vi "Traps-10-06-2017.vi"(0 "d0Trap1":fxp<+/-,18,18> format="%.16g", 1 "heizenTrap1":bool, 2 "U_SPTrap1":fxp<+/-,26,5> format="%.23g", 3 "->Register":u32, 5 "d1Trap1":fxp<+/-,21,21> format="%.16g", 7 "Warten(uSec)":u16=5000, 9 "d0Trap2":fxp<+/-,18,18> format="%.16g", 11 "d1Trap2":fxp<+/-,21,21> format="%.16g", 12 "heizenTrap2":bool, 13 "U_SPTrap2":fxp<+/-,26,5> format="%.23g") -> (4 "U_MWTrap1":fxp<+/-,26,5> format="%.23g", 14 "Register->":u32, 15 "U_MWTrap2":fxp<+/-,26,5> format="%.23g")   [LabVIEW 2010]
uses:
  <vilib>/eio/EIONode/EIONode.xnode
  <vilib>/rvi/eio/nirviEIOImplementation/nirviEIOImplementation.xnode
  <vilib>/rvi/eio/common/nirviEmuClasses.ctl
  <vilib>/rvi/FXPMathLib/FxpAdd/XNode/nifxpmath_Add.xnode
  <vilib>/rvi/FXPMathLib/FxpAdd/subVIs/nifxpmath_Add_SimConfig.ctl
  <vilib>/fxp/LVFixedPointQuantizationPolicyTypeDef.ctl
  <vilib>/fxp/LVFixedPointOverflowPolicyTypeDef.ctl
  <vilib>/rvi/FXPMathLib/FxpDiv/XNode/nifxpmath_Div.xnode
  <vilib>/rvi/FXPMathLib/FxpDiv/subVIs/nifxpmath_Div_SimConfig.ctl
  <vilib>/rvi/FXPMathLib/FxpSub/XNode/nifxpmath_Sub.xnode
  <vilib>/rvi/FXPMathLib/FxpSub/subVIs/nifxpmath_Sub_SimConfig.ctl
  <vilib>/rvi/FXPMathLib/FxpMul/XNode/nifxpmath_Multiplier.xnode
  <vilib>/rvi/FXPMathLib/FxpMul/subVIs/nifxpmath_Mul_SimConfig.ctl
  <vilib>/rvi/eio/common/nirviEmuTemplateMethod_noerrors.vi
  <vilib>/rvi/FXPMathLib/FxpAdd/simVIs/DllFxpAddTemp_sub.vi
  <vilib>/rvi/FXPMathLib/FxpDiv/simVIs/DllFxpDivTemp_sub.vi
  <vilib>/rvi/FXPMathLib/FxpSub/simVIs/DllFxpSubTemp_sub.vi
  <vilib>/rvi/FXPMathLib/FxpMul/simVIs/DllFxpMulTemp_sub.vi
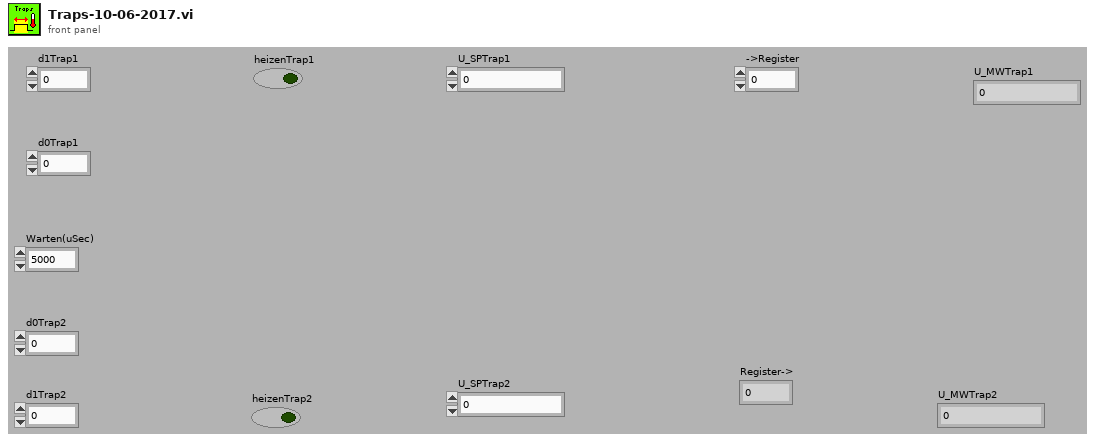
[diagram p1: front panel]
types:
  T1 = typedef "nirviEmuClasses.ctl" = enum16{"IO Read", "IO Write", "Method", "Property Read", "Property Write"}
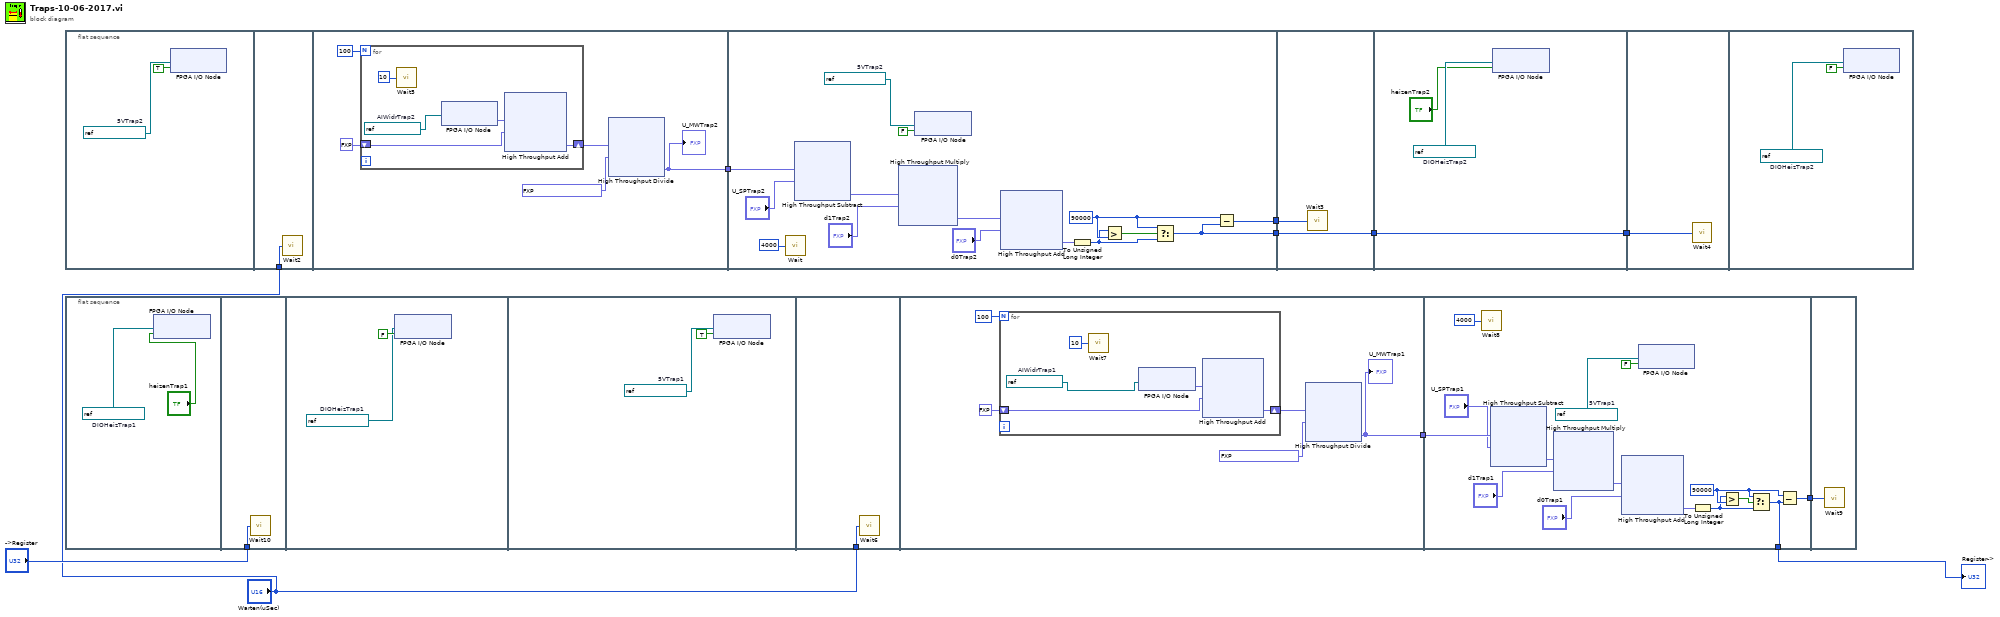
[diagram p0: block diagram]
diagram:
  n1 = flat-sequence {
    tunnel: "Warten(uSec)" -> [w24]
    tunnel: [w25] -> w9
    tunnel: w9 -> [w123]
    tunnel: [w115] -> w8
    tunnel: [w119] -> w7
    tunnel: [w225] -> w6
    tunnel: w8 -> [w225]
    tunnel: w7 -> [w224]
    tunnel: [w228] -> w5
    tunnel: w6 -> [w228]
    tunnel: w5 -> [w240]
    frame #0 {
      w11 = refnum<k21> "Mod6/DIO20"  # 5VTrap2
      n2 = xnode "FPGA I/O Node"("I/O Item"=TRUE, "FPGA I/O In"=w11) -> ()  [unwired: 1 out]
    }
    frame #1 {
      n3 = call "Wait2"("Count(uSec)"=w24) -> ()  [unwired: 1 out]
    }
    frame #2 {
      n4 = for {
        N: 100 -> [_]
        shift-right: [w58] -> w29
        shift-left: fxp<+/-,33,12> 0.0 ("x+y") -> [w59]
        w57 = refnum<k21> "Mod1/AI31"  # AIWidrTrap2
        n5 = call "Wait5"("Count(uSec)"=u8 10) -> ()  [unwired: 1 out]
        n6 = xnode "FPGA I/O Node"("FPGA I/O In"=w57) -> ("I/O Item"=w60:fxp<+/-,26,5>)  [unwired: 1 out]
        n7 = xnode "High Throughput Add"("x"=w60, "y"=w59) -> ("x+y"=w58:fxp<+/-,33,12>)
      }
      n8 = xnode "High Throughput Divide"("x"=w29, "y"=fxp<+/-,8,8> 100.0) -> ("x/y"=w25:fxp<+/-,26,5>)
      "U_MWTrap2" <- w25
    }
    frame #3 {
      w114 = refnum<k21> "Mod6/DIO20"  # 5VTrap2
      w117 = u32 90000 ("x")
      n9 = call "Wait"("Count(uSec)"=u16 4000) -> ()  [unwired: 1 out]
      n10 = xnode "High Throughput Subtract"("x"=w123, "y"="U_SPTrap2") -> ("x-y"=w122:fxp<+/-,26,5>)
      n11 = xnode "High Throughput Multiply"("x"=w122, "y"="d1Trap2") -> ("x*y"=w121:fxp<+/-,18,18>)
      n12 = xnode "FPGA I/O Node"("I/O Item"=FALSE, "FPGA I/O In"=w114) -> ()  [unwired: 1 out]
      n13 = xnode "High Throughput Add"("x"=w121, "y"="d0Trap2") -> ("x+y"=w120:fxp<+/-,18,18>)
      n14 = To Unsigned Long Integer(number=w120) -> (unsigned 32bit integer=w116:u32)
      n15 = Greater?(x=w116, y=w117) -> (0:w118:bool)
      n16 = Select(t=w117, s=w118, f=w116) -> (s? t:f=w115:u32)
      n17 = Subtract(x=w117, y=w115) -> (x-y=w119:u32)
    }
    frame #4 {
      n18 = call "Wait3"("Count(uSec)"=w224) -> ()  [unwired: 1 out]
    }
    frame #5 {
      w227 = refnum<k21> "Mod6/DIO18"  # DIOHeizTrap2
      n19 = xnode "FPGA I/O Node"("I/O Item"="heizenTrap2", "FPGA I/O In"=w227) -> ()  [unwired: 1 out]
    }
    frame #6 {
      n20 = call "Wait4"("Count(uSec)"=w240) -> ()  [unwired: 1 out]
    }
    frame #7 {
      w241 = refnum<k21> "Mod6/DIO18"  # DIOHeizTrap2
      n21 = xnode "FPGA I/O Node"("I/O Item"=FALSE, "FPGA I/O In"=w241) -> ()  [unwired: 1 out]
    }
  }
  n22 = flat-sequence {
    tunnel: "->Register" -> [w267]
    tunnel: "Warten(uSec)" -> [w294]
    tunnel: [w295] -> w4
    tunnel: w4 -> [w393]
    tunnel: [w389] -> w3
    tunnel: [w385] -> w2
    tunnel: w3 -> [w494]
    frame #0 {
      w255 = refnum<k21> "Mod6/DIO19"  # DIOHeizTrap1
      n23 = xnode "FPGA I/O Node"("I/O Item"="heizenTrap1", "FPGA I/O In"=w255) -> ()  [unwired: 1 out]
    }
    frame #1 {
      n24 = call "Wait10"("Count(uSec)"=w267) -> ()  [unwired: 1 out]
    }
    frame #2 {
      w268 = refnum<k21> "Mod6/DIO19"  # DIOHeizTrap1
      n25 = xnode "FPGA I/O Node"("I/O Item"=FALSE, "FPGA I/O In"=w268) -> ()  [unwired: 1 out]
    }
    frame #3 {
      w281 = refnum<k21> "Mod6/DIO21"  # 5VTrap1
      n26 = xnode "FPGA I/O Node"("I/O Item"=TRUE, "FPGA I/O In"=w281) -> ()  [unwired: 1 out]
    }
    frame #4 {
      n27 = call "Wait6"("Count(uSec)"=w294) -> ()  [unwired: 1 out]
    }
    frame #5 {
      n28 = for {
        N: 100 -> [_]
        shift-right: [w328] -> w299
        shift-left: fxp<+/-,33,12> 0.0 ("x+y") -> [w329]
        w327 = refnum<k21> "Mod1/AI30"  # AIWidrTrap1
        n29 = call "Wait7"("Count(uSec)"=u8 10) -> ()  [unwired: 1 out]
        n30 = xnode "FPGA I/O Node"("FPGA I/O In"=w327) -> ("I/O Item"=w330:fxp<+/-,26,5>)  [unwired: 1 out]
        n31 = xnode "High Throughput Add"("x"=w330, "y"=w329) -> ("x+y"=w328:fxp<+/-,33,12>)
      }
      n32 = xnode "High Throughput Divide"("x"=w299, "y"=fxp<+/-,8,8> 100.0) -> ("x/y"=w295:fxp<+/-,26,5>)
      "U_MWTrap1" <- w295
    }
    frame #6 {
      w384 = refnum<k21> "Mod6/DIO21"  # 5VTrap1
      w387 = u32 90000 ("x")
      n33 = call "Wait8"("Count(uSec)"=u16 4000) -> ()  [unwired: 1 out]
      n34 = xnode "High Throughput Subtract"("x"=w393, "y"="U_SPTrap1") -> ("x-y"=w392:fxp<+/-,26,5>)
      n35 = xnode "High Throughput Multiply"("x"=w392, "y"="d1Trap1") -> ("x*y"=w391:fxp<+/-,18,18>)
      n36 = xnode "High Throughput Add"("x"=w391, "y"="d0Trap1") -> ("x+y"=w390:fxp<+/-,18,18>)
      n37 = xnode "FPGA I/O Node"("I/O Item"=FALSE, "FPGA I/O In"=w384) -> ()  [unwired: 1 out]
      n38 = To Unsigned Long Integer(number=w390) -> (unsigned 32bit integer=w386:u32)
      n39 = Greater?(x=w386, y=w387) -> (0:w388:bool)
      n40 = Select(t=w387, s=w388, f=w386) -> (s? t:f=w385:u32)
      n41 = Subtract(x=w387, y=w385) -> (x-y=w389:u32)
    }
    frame #7 {
      n42 = call "Wait9"("Count(uSec)"=w494) -> ()  [unwired: 1 out]
    }
  }
  "Register->" <- w2
